vi "ED_Verify_ACK.vi"(4 "error code":i32, 5 "error code description":string="error code description", 6 "error in (no error)":errorcluster, 9 "connection ID":refnum<k5>) -> (0 "error out":errorcluster, 3 "connection ID out":refnum<k5>)   [LabVIEW 2020, in "CAENels EASY-DRIVER.lvlib"]
uses:
  CAENels EASY-DRIVER.lvlib
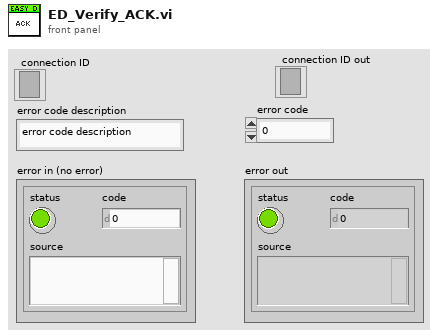
[diagram p1: front panel]
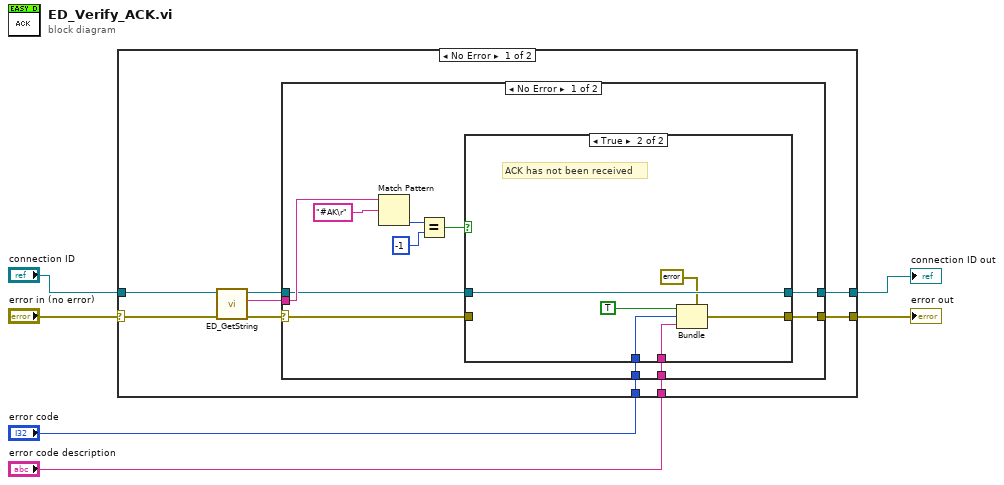
[diagram p0: block diagram]
diagram:
  n1 = case shown="No Error" "error in (no error)" {
    selector: "error in (no error)" -> [w11 w38]
    tunnel: "connection ID" -> [w10 w37]
    tunnel: [w15 w38] -> w4
    tunnel: [w14 w37] -> w3
    tunnel: "error code" -> [w13 _]
    tunnel: "error code description" -> [w12 _]
    frame No Error {
      n2 = call "ED_GetString.vi"("error in"=w11, "connection ID in"=w10) -> ("error out"=w9:errorcluster, "String"=w8:string, "connection ID out"=w7:refnum<k5>)  [unwired: 3 in]
      n3 = case shown="No Error" w9 {
        selector: w9 -> [w21 w36]
        tunnel: [w20 w36] -> w15
        tunnel: [w18 w35] -> w14
        tunnel: w7 -> [w19 w35]
        tunnel: w8 -> [w25 _]
        tunnel: w13 -> [w17 _]
        tunnel: w12 -> [w16 _]
        frame No Error {
          n4 = Match Pattern(string=w25, regular expression="#AK\r") -> (offset past match=w24:i32)  [unwired: 4 out]
          n5 = Equal?(x=w24, y=-1) -> (x = y?=w22:bool)
          n6 = case shown="True" w22 {
            tunnel: [w28 w33] -> w20
            tunnel: w21 -> [w28 _]
            tunnel: w19 -> [w27 w34]
            tunnel: [w27 w34] -> w18
            tunnel: w17 -> [_ w30]
            tunnel: w16 -> [_ w29]
            frame False {
              # "ACK has been found"
            }
            frame True {
              # "ACK has not been received"
              n7 = Bundle(cluster=errorcluster {"status"=FALSE, "code"=0, "source"=""} ("error in  2"), "status"=TRUE, "code"=w30, "source"=w29) -> (w33:errorcluster)
            }
          }
        }
        frame Error {
        }
      }
    }
    frame Error {
    }
  }
  "error out" <- w4
  "connection ID out" <- w3
